vi "Make VI Param(Read Batch Profile Rsp).vi"(1 "pRsp":T2) -> (0 "Read Batch Profile Rsp":T1)   [LabVIEW 2015, in "KEYENCE LJ-X8000A.lvlib"]
uses:
  KEYENCE LJ-X8000A.lvlib
  Public/Clusters/Read Batch Profile Rsp.ctl
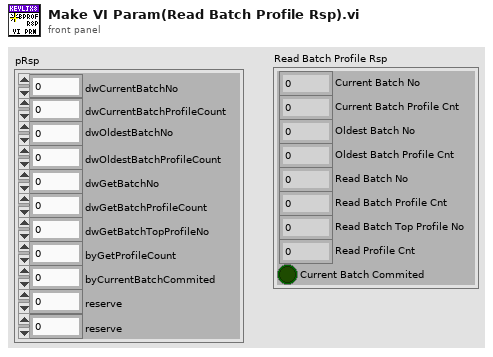
[diagram p1: front panel]
types:
  T1 = typedef "KEYENCE LJ-X8000A.lvlib/Read Batch Profile Rsp.ctl" = cluster{"Current Batch No":u32, "Current Batch Profile Cnt":u32, "Oldest Batch No":u32, "Oldest Batch Profile Cnt":u32, "Read Batch No":u32, "Read Batch Profile Cnt":u32, "Read Batch Top Profile No":u32, "Read Profile Cnt":u32, "Current Batch Commited":bool}
  T2 = cluster{"dwCurrentBatchNo":u32, "dwCurrentBatchProfileCount":u32, "dwOldestBatchNo":u32, "dwOldestBatchProfileCount":u32, "dwGetBatchNo":u32, "dwGetBatchProfileCount":u32, "dwGetBatchTopProfileNo":u32, "byGetProfileCount":u8, "byCurrentBatchCommited":u8, "reserve":u8, "reserve":u8}
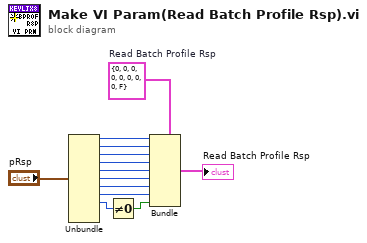
[diagram p0: block diagram]
diagram:
  w2 = T1 {"Current Batch No"=0, "Current Batch Profile Cnt"=0, "Oldest Batch No"=0, "Oldest Batch Profile Cnt"=0, "Read Batch No"=0, "Read Batch Profile Cnt"=0, "Read Batch Top Profile No"=0, "Read Profile Cnt"=0, "Current Batch Commited"=FALSE}  # Read Batch Profile Rsp
  n1 = Unbundle("pRsp") -> ("dwCurrentBatchNo"=w13:u32, "dwCurrentBatchProfileCount"=w12:u32, "dwOldestBatchNo"=w11:u32, "dwOldestBatchProfileCount"=w10:u32, "dwGetBatchNo"=w9:u32, "dwGetBatchProfileCount"=w8:u32, "dwGetBatchTopProfileNo"=w7:u32, "byGetProfileCount"=w6:u8, "byCurrentBatchCommited"=w5:u8)  [unwired: 2 out]
  n2 = Not Equal To 0?(x=w5) -> (x != 0?=w4:bool)
  n3 = Bundle(cluster=w2, "Current Batch No"=w13, "Current Batch Profile Cnt"=w12, "Oldest Batch No"=w11, "Oldest Batch Profile Cnt"=w10, "Read Batch No"=w9, "Read Batch Profile Cnt"=w8, "Read Batch Top Profile No"=w7, "Read Profile Cnt"=w6, "Current Batch Commited"=w4) -> (→"Read Batch Profile Rsp":T1)
